vi "Write COM Port.vi"(8 "error in (no error)":errorcluster, 10 "COM Port":refnum<visa-resource-name>, 11 "H3611i in":refnum<class "H3611i.lvclass">) -> (0 "error out":errorcluster, 3 "H3611i out":refnum<class "H3611i.lvclass">)   [LabVIEW 2017, in "Sensors.lvlib" / "H3611i.lvclass"]
uses:
  H3611i.lvclass
  H3611i.lvclass/H3611i.ctl
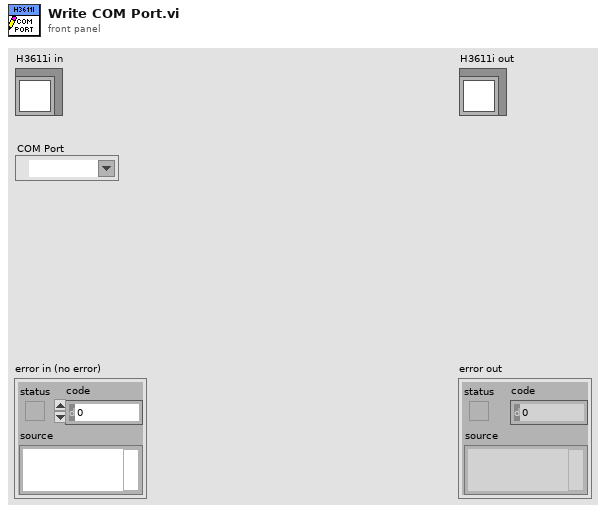
[diagram p1: front panel]
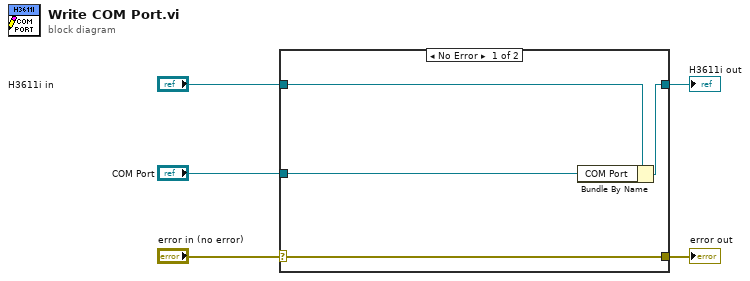
[diagram p0: block diagram]
diagram:
  n1 = case shown="No Error" "error in (no error)" {
    selector: "error in (no error)" -> [w9 w10]
    tunnel: [w9 w10] -> w4
    tunnel: [w7 w11] -> w2
    tunnel: "H3611i in" -> [w8 w11]
    tunnel: "COM Port" -> [w6 _]
    frame No Error {
      n2 = Bundle By Name(cluster=w8, "COM Port"=w6) -> (w7:refnum<class "H3611i.lvclass">)
    }
    frame Error {
    }
  }
  "error out" <- w4
  "H3611i out" <- w2
